vi "FormatDMAelement_2_single_elenet.vi"(8 "valid in":bool, 11 "Data in":fxp<+/-,16,14>[](array[numeric])=[0.0, 0.0, 0.0, 0.0]) -> (0 "valid out":bool, 3 "Element":u64)   [LabVIEW 2013]
uses:
  <vilib>/rvi/FXPMathLib/FxpInterpret/XNode/nifxpmath_Interpret.xnode
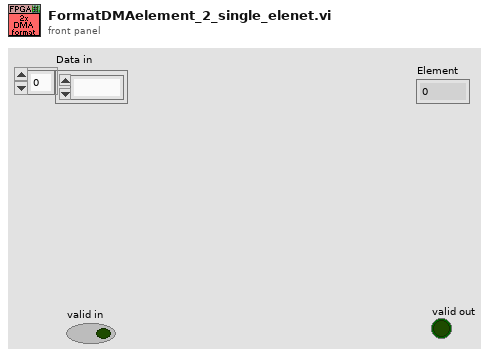
[diagram p1: front panel]
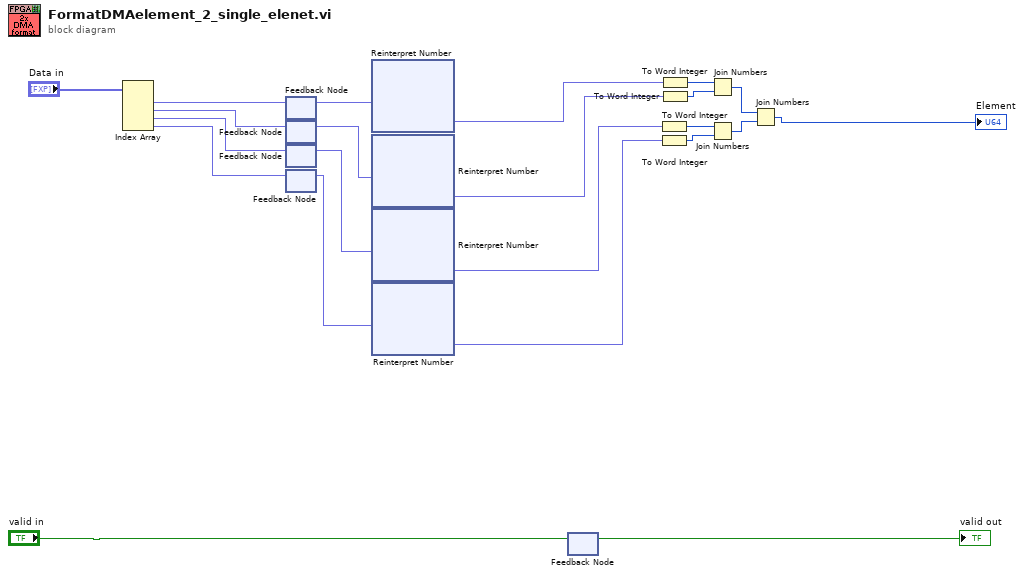
[diagram p0: block diagram]
diagram:
  n1 = Index Array(array="Data in") -> (element #1=w19:fxp<+/-,16,14>, element #2=w18:fxp<+/-,16,14>, element #3=w17:fxp<+/-,16,14>, element #4=w16:fxp<+/-,16,14>)  [unwired: 4 in]
  n2 = feedback #1() -> (w9:fxp<+/-,16,14>)  [unwired: 1 in]
  n3 = feedback-in #1(w19) -> ()
  n4 = feedback #2() -> (w7:fxp<+/-,16,14>)  [unwired: 1 in]
  n5 = feedback-in #2(w18) -> ()
  n6 = feedback #3() -> (w6:fxp<+/-,16,14>)  [unwired: 1 in]
  n7 = feedback-in #3(w17) -> ()
  n8 = feedback #4() -> (w5:fxp<+/-,16,14>)  [unwired: 1 in]
  n9 = feedback-in #4(w16) -> ()
  n10 = xnode "Reinterpret Number"("x"=w9) -> ("y"=w8:fxp<+/-,16,16>)
  n11 = xnode "Reinterpret Number"("x"=w7) -> ("y"=w4:fxp<+/-,16,16>)
  n12 = xnode "Reinterpret Number"("x"=w6) -> ("y"=w3:fxp<+/-,16,16>)
  n13 = xnode "Reinterpret Number"("x"=w5) -> ("y"=w2:fxp<+/-,16,16>)
  n14 = feedback #5() -> (→"valid out":bool)  [unwired: 1 in]
  n15 = feedback-in #5("valid in") -> ()
  n16 = To Word Integer(number=w3) -> (16bit integer=w13:i16)
  n17 = To Word Integer(number=w2) -> (16bit integer=w12:i16)
  n18 = To Word Integer(number=w8) -> (16bit integer=w14:i16)
  n19 = To Word Integer(number=w4) -> (16bit integer=w15:i16)
  n20 = Join Numbers(hi=w14, lo=w15) -> ((hi.lo)=w11:u32)
  n21 = Join Numbers(hi=w13, lo=w12) -> ((hi.lo)=w10:u32)
  n22 = Join Numbers(hi=w11, lo=w10) -> ((hi.lo)=→"Element":u64)
